vi "Evaluate Data.vi"(8 "error in (no error)":errorcluster, 11 "Measurements":dbl[](array[numeric])) -> (0 "error out":errorcluster, 1 "Valid Data?":bool, 2 "Measurement Count":i32, 3 "Average":dbl)   [LabVIEW 2020, in "DMM Msg.lvlib" / "DMM Measurement Data.lvclass"]
doc: "Evaluate the measurements array for average, measurement count and validity."
uses:
  DMM Measurement Data.lvclass
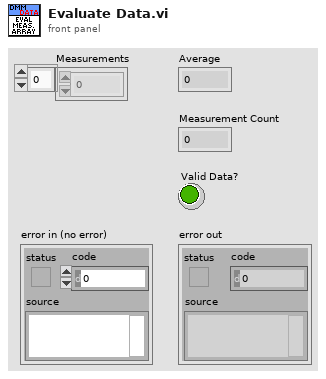
[diagram p1: front panel]
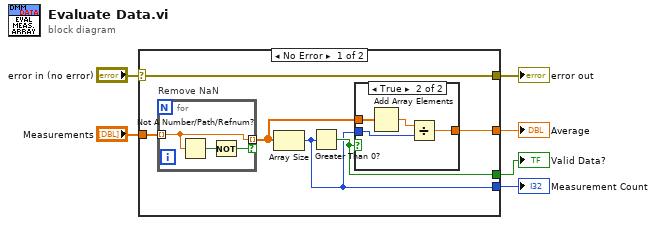
[diagram p0: block diagram]
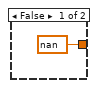
[diagram p2: hidden frame]
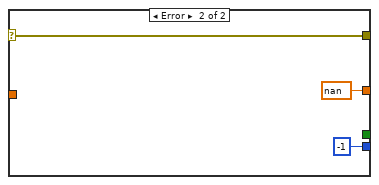
[diagram p3: hidden frame]
diagram:
  n1 = case shown="No Error" "error in (no error)" {
    selector: "error in (no error)" -> [w8 w23]
    tunnel: "Measurements" -> [w11 _]
    tunnel: [w10 nan] -> w5
    tunnel: [w9 _] -> w4
    tunnel: [w8 w23] -> w2
    tunnel: [w7 -1] -> w1
    frame No Error {
      n2 = for "Remove NaN" {
        tunnel: w11 -> [w19] mode=indexing
        tunnel: [w19] -> w12 mode=indexing if=w18
        n3 = Not A Number/Path/Refnum?(number/path/refnum=w19) -> (NaN/Path/Refnum?=w20:bool)
        n4 = Not(x=w20) -> (.not. x?=w18:bool)
      }
      n5 = Array Size(array=w12) -> (size(s)=w7:i32)
      n6 = Greater Than 0?(x=w7) -> (x > 0?=w9:bool)
      n7 = case shown="True" w9 {
        tunnel: w7 -> [_ w17]
        tunnel: w12 -> [_ w16]
        tunnel: [nan w15] -> w10
        frame False {
        }
        frame True {
          n8 = Add Array Elements(numeric array=w16) -> (sum=w14:dbl)
          n9 = Divide(x=w14, y=w17) -> (x/y=w15:dbl)
        }
      }
    }
    frame Error {
    }
  }
  "Valid Data?" <- w4
  "Average" <- w5
  "error out" <- w2
  "Measurement Count" <- w1
